vi "util-address-to-string.vi"(10 "ADDR":T1 format="%04d") -> (2 "str(ADDR)":string)   [LabVIEW 2024]
uses:
  controls/type.address.ctl
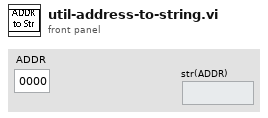
[diagram p1: front panel]
types:
  T1 = typedef "type.address.ctl" = u16
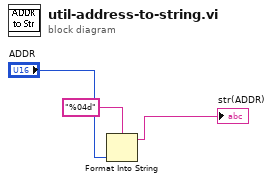
[diagram p0: block diagram]
diagram:
  n1 = Format Into String(format string="%04d", "ADDR") -> (resulting string=→"str(ADDR)":string)  [unwired: 2 in, 1 out]
